vi "Immediate Histogram Trigger.vi"(8 "error in (no error)":errorcluster {"code" format="%.0x"}, 10 "Channel Name (1)":string="1", 11 "VISA resource name":refnum<visa-resource-name>) -> (0 "error out":errorcluster {"code" format="%.0x"}, 3 "VISA resource name out":refnum<visa-resource-name>)   [LabVIEW 2016, in "Agilent N6700 Series.lvlib"]
doc: "Sends an immediate trigger signal to the histogram current measurement data logger. This will trigger the histogram measurement regardless of the selected trigger source.\n\n<b>Notes:</b>\n(1) The histogram must be initiated before triggered.\n(2) This VI only applies to models N6781A and N6782A that have the Data Logger function installed.\n(3) This VI only applies to the N6705B and N6705C DC Power Analyzer."
uses:
  <instrlib>/Agilent N6700 Series/Agilent N6700 Series.lvlib
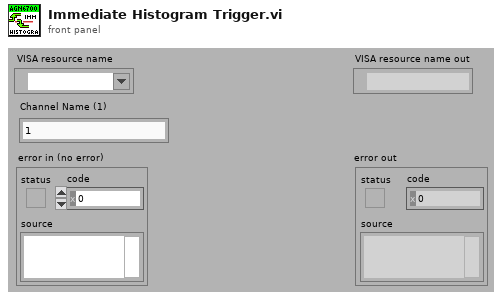
[diagram p1: front panel]
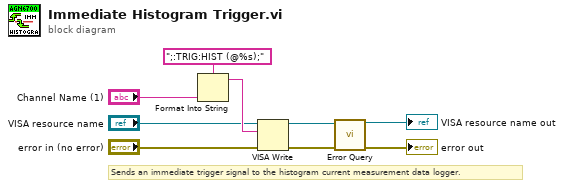
[diagram p0: block diagram]
diagram:
  # "Sends an immediate trigger signal to the histogram current measurement data logger."
  n1 = Format Into String(format string=";:TRIG:HIST (@%s);", "Channel Name (1)") -> (resulting string=w9:string)  [unwired: 2 in, 1 out]
  n2 = VISA Write(VISA resource name="VISA resource name", write buffer=w9, error in (no error)="error in (no error)") -> (VISA resource name out=w2:refnum<visa-resource-name>, error out=w1:errorcluster)  [unwired: 1 out]
  n3 = call <instrlib>:"Error Query.vi"("VISA resource name"=w2, "error in (no error)"=w1) -> ("VISA resource name out"=→"VISA resource name out":refnum<visa-resource-name>, "error out"=→"error out":errorcluster)  [unwired: 10 in, 2 out]
